vi "MW Power sweep contrastvi.vi"() -> ()   [LabVIEW 2012]
uses:
  <vilib>/Analysis/1siggen.llb/Ramp Pattern by Samples.vi
  <vilib>/Utility/file.llb/Write To Spreadsheet File (DBL).vi
  <vilib>/Analysis/NI_AALBase.lvlib
panel:
  out "XY Graph":cluster{"Y":dbl[], "Y":dbl[]}[](graph)
  in  "Channel":bool=TRUE
  in  "leveling file":path=path "C:/Users/Ouyang Group/Documents/Data/8-5-16/wavetek power calibration double sweep -4dbm interp 3"
  in  "leveling":bool
  out "COM Error":bool
  out "Level":bool
  in  "f":dbl
  in  "file path (dialog if empty)":path
  in  "p start":dbl format="%0.2f"
  in  "p end":dbl=1.0 format="%0.2f"
  in  "p samples":i32=128
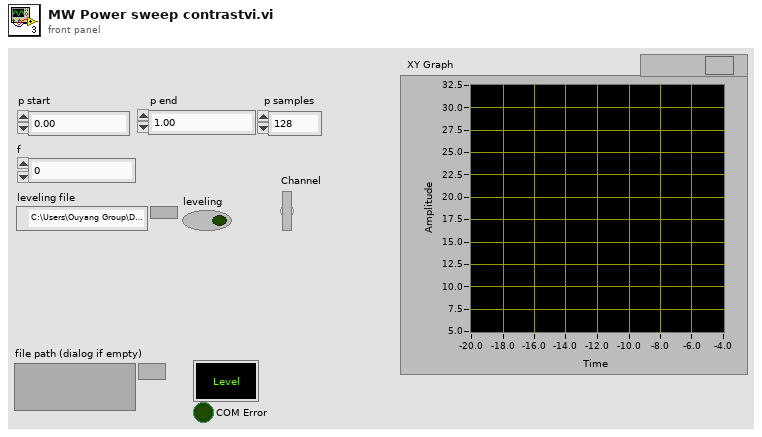
[diagram p1: front panel]
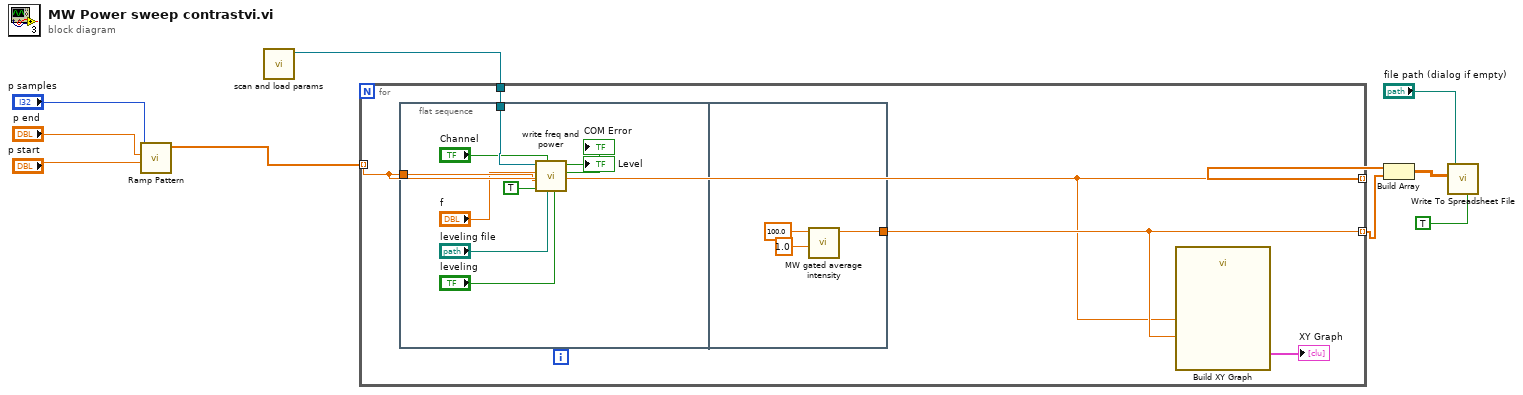
[diagram p0: block diagram]
diagram:
  n1 = call-poly <vilib>:"Ramp Pattern.vi"("start"="p start", "end"="p end", "samples"="p samples") -> ("Ramp Pattern"=w5:dbl[])  [unwired: 7 in, 1 out]
  n2 = call "scan and load params.vi"() -> ("Serial Port Select"=w2:refnum<visa-resource-name>)  [unwired: 9 out]
  n3 = for {
    tunnel: w5 -> [w11] mode=indexing
    tunnel: [w11] -> w3 mode=indexing
    tunnel: w2 -> [w14]
    tunnel: [w12] -> w1 mode=indexing
    n4 = flat-sequence {
      tunnel: w11 -> [w16]
      tunnel: w14 -> [w23]
      tunnel: [w24] -> w12
      frame #0 {
        n5 = call "write freq and power.vi"("leveling"="leveling", "leviling file"="leveling file", "Channel"="Channel", "RF On"=TRUE, "p (dbm)"=w16, "f (Hz)"="f", "Serial Port Select"=w23) -> ("COM Error"=→"COM Error":bool, "Level"=→"Level":bool)  [unwired: 3 in]
      }
      frame #1 {
        n6 = call "MW gated average intensity.vi"("Time"=1.0, "rate"=100.0) -> ("Contrast (%)"=w24:dbl)  [unwired: 9 in]
      }
    }
    n7 = call "Build XY Graph"("Y Input"=w12, "X Input"=w11) -> ("XY Graph"=→"XY Graph":cluster{"Y":dbl[], "Y":dbl[]}[])  [unwired: 3 in, 6 out]
  }
  n8 = Build Array(w3, w1) -> (w4:dbl[][])
  n9 = call-poly <vilib>:"Write To Spreadsheet File.vi"("transpose? (no:F)"=TRUE, "2D data"=w4, "file path (dialog if empty)"="file path (dialog if empty)") -> ()  [unwired: 5 in, 1 out]
